vi "AODO-Synchronize Tasks.vi"(0 "Tasks In":T1[](array[typedef]), 7 "external trig":bool, 9 "Trig Src":string, 11 "error in (no error)":errorcluster) -> (4 "Tasks Out":T1[](array[typedef]), 8 "Sync Task":refnum<k21>, 10 "Start Trigger Terminal":string, 15 "error out":errorcluster)   [LabVIEW 2020]
uses:
  Typedefs/AODO-Task Specification.ctl
  <vilib>/DAQmx/configure/trigger.llb/DAQmx Start Trigger (Digital Edge).vi
  <resource>/objmgr/daqmx.rc
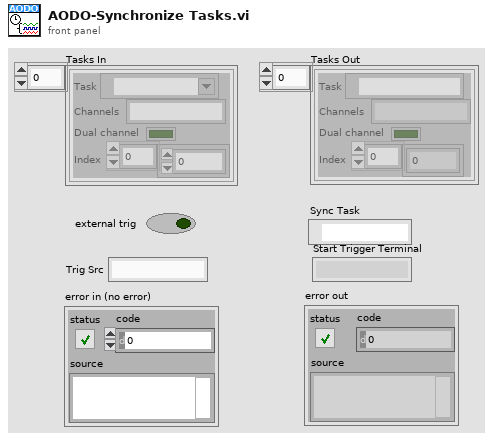
[diagram p1: front panel]
types:
  T1 = typedef "AODO-Task Specification.ctl" = cluster{"Task":refnum<k21>, "Channels":string, "Dual channel":bool, "Index":i32[]}
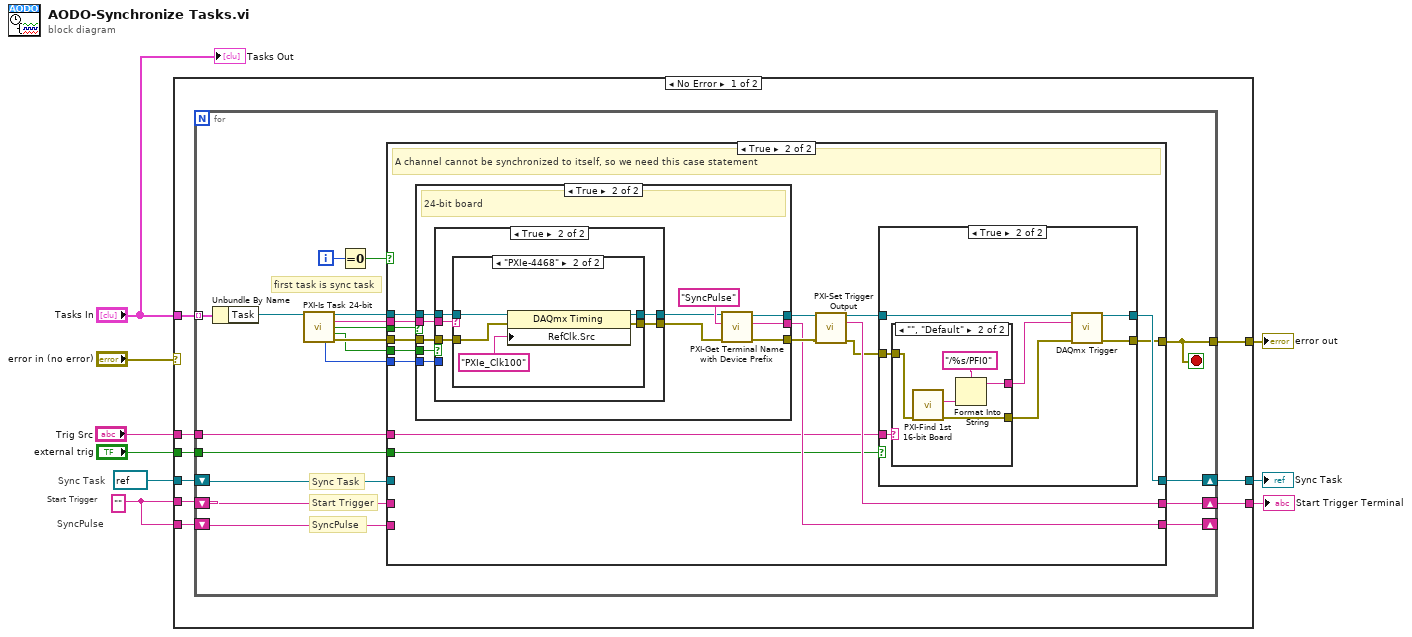
[diagram p0: block diagram]
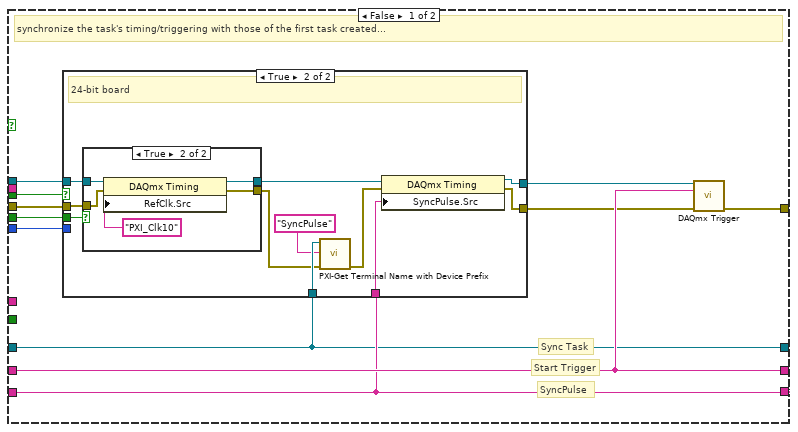
[diagram p2: hidden frame]
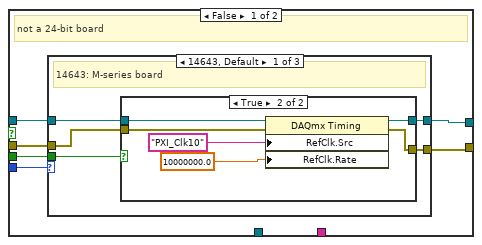
[diagram p3: hidden frame]
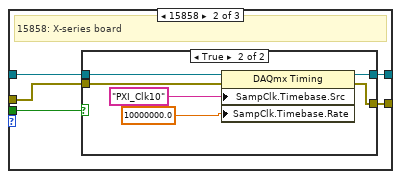
[diagram p5: hidden frame]
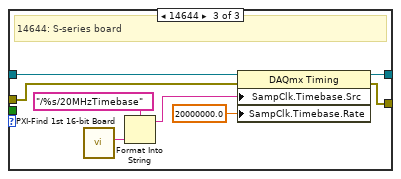
[diagram p7: hidden frame]
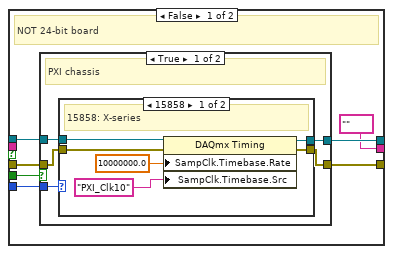
[diagram p11: hidden frame]
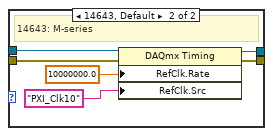
[diagram p12: hidden frame]
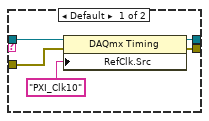
[diagram p15: hidden frame]
diagram:
  w2 = ""
  # "SyncPulse"
  # "Start Trigger"
  # "Sync Task"
  n1 = case shown="No Error" "error in (no error)" {
    selector: "error in (no error)" -> [_ w193]
    tunnel: refnum<k21> refnum ("task out") -> [w18 _]
    tunnel: w2 -> [w17 _]
    tunnel: w2 -> [w16 _]
    tunnel: "Tasks In" -> [w15 _]
    tunnel: [w14 w193] -> w6
    tunnel: [w13 _] -> w5
    tunnel: "external trig" -> [w12 _]
    tunnel: "Trig Src" -> [w11 _]
    tunnel: [w10 _] -> w1
    frame No Error {
      n2 = for {
        shift-right: [w37] -> w13
        shift-left: w18 -> [w25]
        shift-right: [w35] -> w10
        shift-left: w17 -> [w24]
        shift-right: [w34] -> _
        shift-left: w16 -> [w23]
        tunnel: [w29] -> w14
        tunnel: w15 -> [w27] mode=indexing
        tunnel: w12 -> [w22]
        tunnel: w11 -> [w21]
        i -> [w36]
        stop <- w29 stop-if-true
        # "SyncPulse"
        # "Start Trigger"
        # "Sync Task"
        # "first task is sync task"
        n3 = Unbundle By Name(w27) -> ("Task"=w26:refnum<k21>)
        n4 = call "PXI-Is Task 24-bit.vi"("task"=w26) -> ("task out"=w31:refnum<k21>, "Product Type"=w19:string, "is 24bit?"=w28:bool, "PXI?"=w20:bool, "Product Category"=w30:i32, "error out"=w32:errorcluster)  [unwired: 9 in]
        n5 = Equal To 0?(x=w36) -> (x = 0?=w33:bool)
        n6 = case shown="True" w33 {
          tunnel: w32 -> [w46 w117]
          tunnel: [w48 w110] -> w29
          tunnel: [w40 w111] -> w37
          tunnel: w25 -> [w40 _]
          tunnel: [w47 w119] -> w35
          tunnel: w24 -> [w47 _]
          tunnel: [w45 w120] -> w34
          tunnel: w23 -> [w45 _]
          tunnel: w31 -> [w41 w118]
          tunnel: w28 -> [w42 w116]
          tunnel: w30 -> [w39 w115]
          tunnel: w20 -> [w38 w114]
          tunnel: w22 -> [_ w109]
          tunnel: w21 -> [_ w108]
          tunnel: w19 -> [_ w107]
          frame False {
            # "SyncPulse"
            # "Start Trigger"
            # "Sync Task"
            # "synchronize the task's timing/triggering with those of the first task created..."
            n7 = case shown="True" w42 {
              tunnel: [w52 w99] -> w44
              tunnel: [w53 w98] -> w43
              tunnel: w40 -> [_ w97]
              tunnel: w46 -> [w50 w96]
              tunnel: w45 -> [_ w95]
              tunnel: w41 -> [w51 w90]
              tunnel: w39 -> [w54 _]
              tunnel: w38 -> [w49 w89]
              frame False {
                # "not a 24-bit board"
                n8 = case shown="14643, Default" w54 {
                  tunnel: [w59 w72 w88] -> w52
                  tunnel: [w58 w71 w87] -> w53
                  tunnel: w51 -> [w57 w70 w85]
                  tunnel: w50 -> [w56 w69 w84]
                  tunnel: w49 -> [w55 w68 _]
                  frame 14643, Default {
                    # "14643: M-series board"
                    n9 = case shown="True" w55 {
                      tunnel: [w61 w67] -> w59
                      tunnel: [w60 w66] -> w58
                      tunnel: w57 -> [w61 w63]
                      tunnel: w56 -> [w60 w62]
                      frame False {
                      }
                      frame True {
                        n10 = property class="DAQmx Timing"(reference=w63, error in=w62, "RefClk.Src"="PXI_Clk10", "RefClk.Rate"=10000000.0) -> (reference out=w67:refnum<k21>, error out=w66:errorcluster)
                      }
                    }
                  }
                  frame 15858 {
                    # "15858: X-series board"
                    n11 = case shown="True" w68 {
                      tunnel: [w74 w80] -> w72
                      tunnel: [w73 w79] -> w71
                      tunnel: w70 -> [w74 w76]
                      tunnel: w69 -> [w73 w75]
                      frame False {
                      }
                      frame True {
                        n12 = property class="DAQmx Timing"(reference=w76, error in=w75, "SampClk.Timebase.Src"="PXI_Clk10" ("RefClk.Src"), "SampClk.Timebase.Rate"=10000000.0) -> (reference out=w80:refnum<k21>, error out=w79:errorcluster)
                      }
                    }
                  }
                  frame 14644 {
                    # "14644: S-series board"
                    n13 = call "PXI-Find 1st 16-bit Board.vi"() -> ("DAQmx Device Name"=w81:tag)  [unwired: 9 in, 2 out]
                    n14 = Format Into String(format string="/%s/20MHzTimebase", w81) -> (resulting string=w82:string)  [unwired: 2 in, 1 out]
                    n15 = property class="DAQmx Timing"(reference=w85, error in=w84, "SampClk.Timebase.Src"=w82, "SampClk.Timebase.Rate"=20000000.0) -> (reference out=w88:refnum<k21>, error out=w87:errorcluster)
                  }
                }
              }
              frame True {
                # "24-bit board"
                n16 = case shown="True" w89 {
                  tunnel: w96 -> [w100 w106]
                  tunnel: [w100 w105] -> w92
                  tunnel: [w101 w104] -> w91
                  tunnel: w90 -> [w101 w103]
                  frame False {
                  }
                  frame True {
                    n17 = property class="DAQmx Timing"(reference=w103, error in=w106, "RefClk.Src"="PXI_Clk10") -> (reference out=w104:refnum<k21>, error out=w105:errorcluster)
                  }
                }
                n18 = call "PXI-Get Terminal Name with Device Prefix.vi"("error in (no error)"=w92, "Local Terminal Name"="SyncPulse", "task/channels in"=w97) -> ("error out"=w93:errorcluster)  [unwired: 6 in, 2 out]
                n19 = property class="DAQmx Timing"(reference=w91, error in=w93, "SyncPulse.Src"=w95) -> (reference out=w99:refnum<k21>, error out=w98:errorcluster)
              }
            }
            n20 = call-poly <vilib>:"DAQmx Trigger.vi"("task/channels in"=w44, "source"=w47, "error in"=w43) -> ("error out"=w48:errorcluster)  [unwired: 11 in, 1 out]
          }
          frame True {
            # "A channel cannot be synchronized to itself, so we need this case statement"
            n21 = case shown="True" w116 {
              tunnel: [w144 w175] -> w121
              tunnel: w118 -> [w145 w169]
              tunnel: [w143 w174] -> w122
              tunnel: w117 -> [w142 w168]
              tunnel: [tag "" ("Terminal Name with Device Prefix") w173] -> w120
              tunnel: w115 -> [w139 w166]
              tunnel: w114 -> [w140 w167]
              tunnel: w107 -> [_ w165]
              frame False {
                # "NOT 24-bit board"
                n22 = case shown="True" w140 {
                  tunnel: w145 -> [w150 w164]
                  tunnel: [w149 w164] -> w144
                  tunnel: [w148 w163] -> w143
                  tunnel: w142 -> [w147 w163]
                  tunnel: w139 -> [w146 _]
                  frame True {
                    # "PXI chassis"
                    n23 = case shown="15858" w146 {
                      tunnel: w150 -> [w156 w162]
                      tunnel: [w155 w161] -> w149
                      tunnel: [w154 w160] -> w148
                      tunnel: w147 -> [w153 w159]
                      frame 15858 {
                        # "15858: X-series"
                        n24 = property class="DAQmx Timing"(reference=w156, error in=w153, "SampClk.Timebase.Rate"=10000000.0, "SampClk.Timebase.Src"="PXI_Clk10" ("RefClk.Src")) -> (reference out=w155:refnum<k21>, error out=w154:errorcluster)
                      }
                      frame 14643, Default {
                        # "14643: M-series"
                        n25 = property class="DAQmx Timing"(reference=w162, error in=w159, "RefClk.Rate"=10000000.0, "RefClk.Src"="PXI_Clk10") -> (reference out=w161:refnum<k21>, error out=w160:errorcluster)
                      }
                    }
                  }
                  frame False {
                    # "NOT PXI chassis"
                  }
                }
              }
              frame True {
                # "24-bit board"
                n26 = case shown="True" w167 {
                  tunnel: [w177 w182] -> w171
                  tunnel: [w176 w181] -> w170
                  tunnel: w169 -> [w177 w180]
                  tunnel: w168 -> [w176 w179]
                  tunnel: w166 -> [_ _]
                  tunnel: w165 -> [_ w178]
                  frame False {
                  }
                  frame True {
                    n27 = case shown="\"PXIe-4468\"" w178 {
                      tunnel: [w187 w192] -> w182
                      tunnel: [w186 w191] -> w181
                      tunnel: w180 -> [w185 w190]
                      tunnel: w179 -> [w184 w189]
                      frame Default {
                        n28 = property class="DAQmx Timing"(reference=w185, error in=w184, "RefClk.Src"="PXI_Clk10") -> (reference out=w187:refnum<k21>, error out=w186:errorcluster)
                      }
                      frame "PXIe-4468" {
                        n29 = property class="DAQmx Timing"(reference=w190, error in=w189, "RefClk.Src"="PXIe_Clk100") -> (reference out=w192:refnum<k21>, error out=w191:errorcluster)
                      }
                    }
                  }
                }
                n30 = call "PXI-Get Terminal Name with Device Prefix.vi"("error in (no error)"=w170, "Local Terminal Name"="SyncPulse", "task/channels in"=w171) -> ("error out"=w174:errorcluster, "Terminal Name with Device Prefix"=w173:string, "task out"=w175:refnum<k21>)  [unwired: 6 in]
              }
            }
            n31 = call "PXI-Set Trigger Output.vi"("Task in"=w121, "error in (no error)"=w122) -> ("Task out"=w112:refnum<k21>, "Trigger Terminal"=w119:string, "error out"=w113:errorcluster)  [unwired: 11 in]
            n32 = case shown="True" w109 {
              tunnel: [w123 w131] -> w110
              tunnel: w112 -> [w124 w130]
              tunnel: w113 -> [w123 w128]
              tunnel: [w124 w129] -> w111
              tunnel: w108 -> [_ w125]
              frame False {
              }
              frame True {
                n33 = case shown="\"\", \"Default\"" w125 {
                  selector: w125 -> [w133 _]
                  tunnel: w128 -> [w132 w138]
                  tunnel: [w132 w137] -> w127
                  tunnel: [w133 w134] -> w126
                  frame "else", Default {
                  }
                  frame "", "Default" {
                    n34 = call "PXI-Find 1st 16-bit Board.vi"("error in (no error)"=w138) -> ("error out"=w137:errorcluster, "DAQmx Device Name"=w136:tag)  [unwired: 8 in, 1 out]
                    n35 = Format Into String(format string="/%s/PFI0", w136) -> (resulting string=w134:string)  [unwired: 2 in, 1 out]
                  }
                }
                n36 = call-poly <vilib>:"DAQmx Trigger.vi"("task/channels in"=w130, "source"=w126, "error in"=w127) -> ("task out"=w129:refnum<k21>, "error out"=w131:errorcluster)  [unwired: 11 in]
              }
            }
          }
        }
      }
    }
    frame Error {
    }
  }
  "error out" <- w6
  "Sync Task" <- w5
  "Start Trigger Terminal" <- w1
  "Tasks Out" <- "Tasks In"
